vi "mandelbrot.vi"() -> ()   [LabVIEW 2012]
panel:
  out "mandelbrot set":dbl[][](graph)
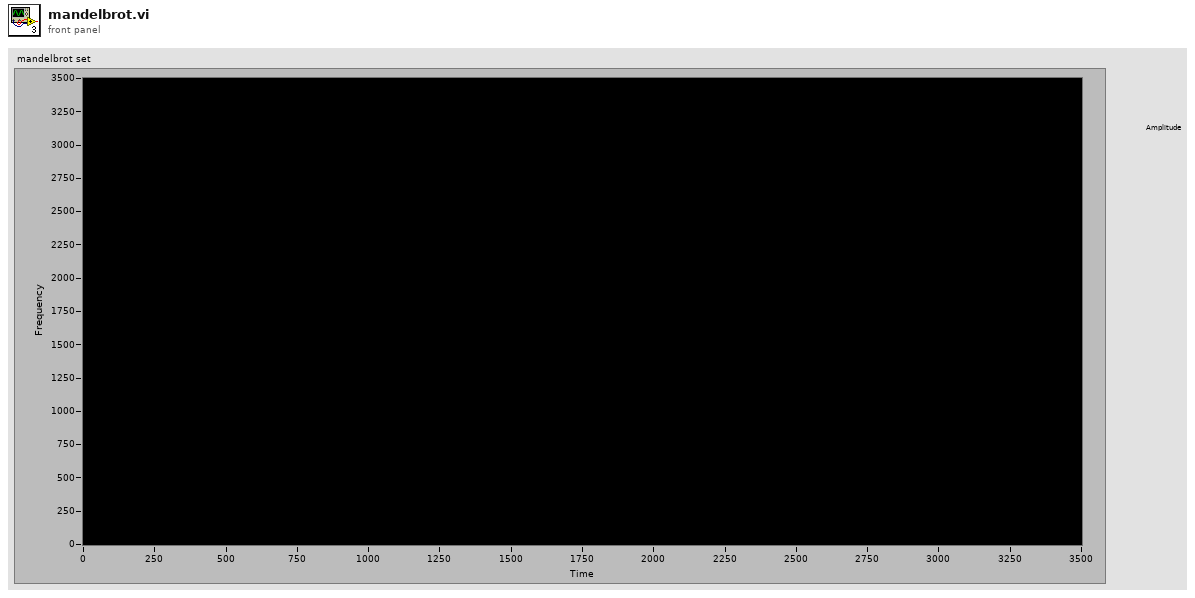
[diagram p1: front panel]
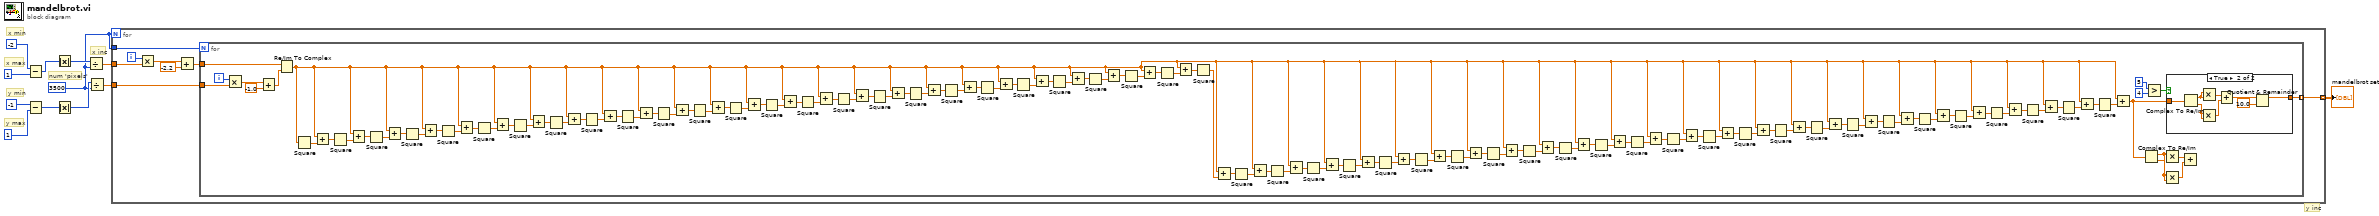
[diagram p0: block diagram]
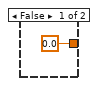
[diagram p2: hidden frame]
diagram:
  w2 = 3500
  # "y inc"
  # "x inc"
  # "num 'pixels'"
  # "y max"
  # "y min"
  # "x max"
  # "x min"
  n1 = Subtract(x=-2, y=1) -> (x-y=w10:i32)
  n2 = Subtract(x=-1, y=1) -> (x-y=w8:i32)
  n3 = Absolute Value(x=w10) -> (abs(x)=w9:i32)
  n4 = Absolute Value(x=w8) -> (abs(x)=w7:i32)
  n5 = Divide(x=w9, y=w2) -> (x/y=w4:dbl)
  n6 = Divide(x=w7, y=w2) -> (x/y=w3:dbl)
  n7 = for {
    N: w2 -> [_]
    tunnel: w4 -> [w19]
    tunnel: w3 -> [w18]
    tunnel: w2 -> [w17]
    tunnel: [w16] -> w1 mode=indexing
    i -> [w20]
    n8 = Multiply(x=w20, y=w19) -> (x*y=w14:dbl)
    n9 = Add(x=w14, y=-2.2) -> (x+y=w15:dbl)
    n10 = for {
      N: w17 -> [_]
      tunnel: w18 -> [w136]
      tunnel: w15 -> [w135]
      tunnel: [w26] -> w16 mode=indexing
      i -> [w137]
      n11 = Multiply(x=w137, y=w136) -> (x*y=w23:dbl)
      n12 = Add(x=w23, y=-1.0) -> (x+y=w22:dbl)
      n13 = Re/Im To Complex(1:w22, 2:w135) -> (0:w25:cdb)
      n14 = Square(x=w25) -> (x^2=w134:cdb)
      n15 = Add(x=w25, y=w134) -> (x+y=w126:cdb)
      n16 = Square(x=w126) -> (x^2=w127:cdb)
      n17 = Add(x=w25, y=w127) -> (x+y=w76:cdb)
      n18 = Square(x=w76) -> (x^2=w125:cdb)
      n19 = Add(x=w25, y=w125) -> (x+y=w75:cdb)
      n20 = Square(x=w75) -> (x^2=w124:cdb)
      n21 = Add(x=w25, y=w124) -> (x+y=w74:cdb)
      n22 = Square(x=w74) -> (x^2=w123:cdb)
      n23 = Add(x=w25, y=w123) -> (x+y=w73:cdb)
      n24 = Square(x=w73) -> (x^2=w106:cdb)
      n25 = Add(x=w25, y=w106) -> (x+y=w72:cdb)
      n26 = Square(x=w72) -> (x^2=w105:cdb)
      n27 = Add(x=w25, y=w105) -> (x+y=w71:cdb)
      n28 = Square(x=w71) -> (x^2=w96:cdb)
      n29 = Add(x=w25, y=w96) -> (x+y=w70:cdb)
      n30 = Square(x=w70) -> (x^2=w95:cdb)
      n31 = Add(x=w25, y=w95) -> (x+y=w69:cdb)
      n32 = Square(x=w69) -> (x^2=w86:cdb)
      n33 = Add(x=w25, y=w86) -> (x+y=w68:cdb)
      n34 = Square(x=w68) -> (x^2=w85:cdb)
      n35 = Add(x=w25, y=w85) -> (x+y=w67:cdb)
      n36 = Square(x=w67) -> (x^2=w122:cdb)
      n37 = Add(x=w25, y=w122) -> (x+y=w66:cdb)
      n38 = Square(x=w66) -> (x^2=w121:cdb)
      n39 = Add(x=w25, y=w121) -> (x+y=w65:cdb)
      n40 = Square(x=w65) -> (x^2=w120:cdb)
      n41 = Add(x=w25, y=w120) -> (x+y=w64:cdb)
      n42 = Square(x=w64) -> (x^2=w119:cdb)
      n43 = Add(x=w25, y=w119) -> (x+y=w63:cdb)
      n44 = Square(x=w63) -> (x^2=w104:cdb)
      n45 = Add(x=w25, y=w104) -> (x+y=w62:cdb)
      n46 = Square(x=w62) -> (x^2=w103:cdb)
      n47 = Add(x=w25, y=w103) -> (x+y=w61:cdb)
      n48 = Square(x=w61) -> (x^2=w94:cdb)
      n49 = Add(x=w25, y=w94) -> (x+y=w60:cdb)
      n50 = Square(x=w60) -> (x^2=w93:cdb)
      n51 = Add(x=w25, y=w93) -> (x+y=w59:cdb)
      n52 = Square(x=w59) -> (x^2=w84:cdb)
      n53 = Add(x=w25, y=w84) -> (x+y=w58:cdb)
      n54 = Square(x=w58) -> (x^2=w83:cdb)
      n55 = Add(x=w25, y=w83) -> (x+y=w57:cdb)
      n56 = Square(x=w57) -> (x^2=w118:cdb)
      n57 = Add(x=w25, y=w118) -> (x+y=w56:cdb)
      n58 = Square(x=w56) -> (x^2=w117:cdb)
      n59 = Add(x=w25, y=w117) -> (x+y=w55:cdb)
      n60 = Square(x=w55) -> (x^2=w116:cdb)
      n61 = Add(x=w25, y=w116) -> (x+y=w54:cdb)
      n62 = Square(x=w54) -> (x^2=w115:cdb)
      n63 = Add(x=w25, y=w115) -> (x+y=w53:cdb)
      n64 = Square(x=w53) -> (x^2=w102:cdb)
      n65 = Add(x=w25, y=w102) -> (x+y=w52:cdb)
      n66 = Square(x=w52) -> (x^2=w101:cdb)
      n67 = Add(x=w25, y=w101) -> (x+y=w51:cdb)
      n68 = Square(x=w51) -> (x^2=w92:cdb)
      n69 = Add(x=w25, y=w92) -> (x+y=w50:cdb)
      n70 = Square(x=w50) -> (x^2=w91:cdb)
      n71 = Add(x=w25, y=w91) -> (x+y=w49:cdb)
      n72 = Square(x=w49) -> (x^2=w82:cdb)
      n73 = Add(x=w25, y=w82) -> (x+y=w48:cdb)
      n74 = Square(x=w48) -> (x^2=w81:cdb)
      n75 = Add(x=w25, y=w81) -> (x+y=w28:cdb)
      n76 = Square(x=w28) -> (x^2=w114:cdb)
      n77 = Add(x=w25, y=w114) -> (x+y=w47:cdb)
      n78 = Square(x=w47) -> (x^2=w113:cdb)
      n79 = Add(x=w25, y=w113) -> (x+y=w46:cdb)
      n80 = Square(x=w46) -> (x^2=w112:cdb)
      n81 = Add(x=w25, y=w112) -> (x+y=w45:cdb)
      n82 = Square(x=w45) -> (x^2=w111:cdb)
      n83 = Add(x=w25, y=w111) -> (x+y=w44:cdb)
      n84 = Square(x=w44) -> (x^2=w100:cdb)
      n85 = Add(x=w25, y=w100) -> (x+y=w43:cdb)
      n86 = Square(x=w43) -> (x^2=w99:cdb)
      n87 = Add(x=w25, y=w99) -> (x+y=w42:cdb)
      n88 = Square(x=w42) -> (x^2=w90:cdb)
      n89 = Add(x=w25, y=w90) -> (x+y=w41:cdb)
      n90 = Square(x=w41) -> (x^2=w89:cdb)
      n91 = Add(x=w25, y=w89) -> (x+y=w40:cdb)
      n92 = Square(x=w40) -> (x^2=w80:cdb)
      n93 = Add(x=w25, y=w80) -> (x+y=w39:cdb)
      n94 = Square(x=w39) -> (x^2=w79:cdb)
      n95 = Add(x=w25, y=w79) -> (x+y=w38:cdb)
      n96 = Square(x=w38) -> (x^2=w110:cdb)
      n97 = Add(x=w25, y=w110) -> (x+y=w37:cdb)
      n98 = Square(x=w37) -> (x^2=w109:cdb)
      n99 = Add(x=w25, y=w109) -> (x+y=w36:cdb)
      n100 = Square(x=w36) -> (x^2=w108:cdb)
      n101 = Add(x=w25, y=w108) -> (x+y=w35:cdb)
      n102 = Square(x=w35) -> (x^2=w107:cdb)
      n103 = Add(x=w25, y=w107) -> (x+y=w34:cdb)
      n104 = Square(x=w34) -> (x^2=w98:cdb)
      n105 = Add(x=w25, y=w98) -> (x+y=w33:cdb)
      n106 = Square(x=w33) -> (x^2=w97:cdb)
      n107 = Add(x=w25, y=w97) -> (x+y=w32:cdb)
      n108 = Square(x=w32) -> (x^2=w88:cdb)
      n109 = Add(x=w25, y=w88) -> (x+y=w31:cdb)
      n110 = Square(x=w31) -> (x^2=w87:cdb)
      n111 = Add(x=w25, y=w87) -> (x+y=w30:cdb)
      n112 = Square(x=w30) -> (x^2=w78:cdb)
      n113 = Add(x=w25, y=w78) -> (x+y=w29:cdb)
      n114 = Square(x=w29) -> (x^2=w77:cdb)
      n115 = Add(x=w25, y=w77) -> (x+y=w27:cdb)
      n116 = Complex To Re/Im(x + iy=w27) -> (x=w132:dbl, y=w133:dbl)
      n117 = Greater?(x=5, y=4) -> (0:w128:bool)
      n118 = Multiply(x=w132, y=w132) -> (x*y=w131:dbl)
      n119 = Multiply(x=w133, y=w133) -> (x*y=w130:dbl)
      n120 = case shown="True" w128 {
        tunnel: [0.0 w139] -> w26
        tunnel: w27 -> [_ w143]
        frame False {
        }
        frame True {
          n121 = Complex To Re/Im(x + iy=w143) -> (x=w141:dbl, y=w146:dbl)
          n122 = Multiply(x=w141, y=w141) -> (x*y=w145:dbl)
          n123 = Multiply(x=w146, y=w146) -> (x*y=w144:dbl)
          n124 = Add(x=w145, y=w144) -> (x+y=w142:dbl)
          n125 = Quotient & Remainder(x=w142, y=10.0) -> (x-y*floor(x/y)=w139:dbl)  [unwired: 1 out]
        }
      }
      n126 = Add(x=w131, y=w130) -> ()  [unwired: 1 out]
    }
  }
  "mandelbrot set" <- w1
